vi "Write configuration.vi"(8 "error in (no error)":errorcluster, 11 "Cascade in":refnum<class "Cascade.lvclass">) -> (0 "error out":errorcluster, 3 "Cascade out":refnum<class "Cascade.lvclass">)   [LabVIEW 2012, in "Cascade.lvclass"]
doc: "Writes the configuration cluster into the configuration file. Configuration file is XML-based. It's name is <component ID>.xml"
uses:
  Cascade.lvclass
  <vilib>/Distrio/Murmex/Murmex/Murmex.lvclass
  Cascade.lvclass/Cascade.ctl
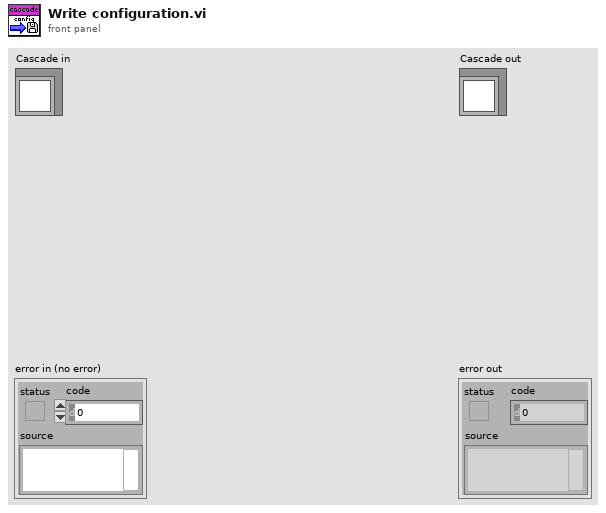
[diagram p1: front panel]
types:
  T1 = typedef "Cascade.lvclass/configuration.ctl" = cluster{"Numeric":dbl}
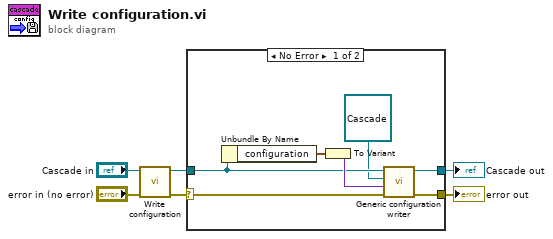
[diagram p0: block diagram]
diagram:
  n1 = call-parent "Write configuration.vi"("error in (no error)"="error in (no error)", "Murmex in"="Cascade in") -> ("error out"=w4:errorcluster, "Murmex out"=w2:refnum<class "Cascade.lvclass">)  [unwired: 8 in]
  n2 = case shown="No Error" w4 {
    selector: w4 -> [w11 w14]
    tunnel: [w10 w14] -> w3
    tunnel: w2 -> [w9 w15]
    tunnel: [w7 w15] -> w1
    frame No Error {
      n3 = Unbundle By Name(w9) -> ("configuration"=w13:T1)
      n4 = To Variant(anything=w13) -> (Variant=w12:variant)
      n5 = call <vilib>:"Generic configuration writer.vi"("error in (no error)"=w11, "configuration"=w12, "inheritance level"=refnum<class "Cascade.lvclass"> refnum ("Cascade.lvclass"), "MurmexBase in"=w9) -> ("error out"=w10:errorcluster, "MurmexBase out"=w7:refnum<class "Cascade.lvclass">)  [unwired: 6 in]
    }
    frame Error {
    }
  }
  "error out" <- w3
  "Cascade out" <- w1
